vi "psk rx.vi"   [LabVIEW 2014]
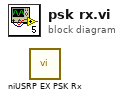
[diagram p0: block diagram]
diagram:
  n1 = call "niUSRP EX PSK Rx.vi"() -> ()  [unwired: 1 in]
